vi "Initialize Sequence.vi"(8 "error in (no error)":errorcluster, 11 "Sequencer in":refnum<class "Sequencer.lvclass">) -> (0 "error out":errorcluster, 3 "Sequencer out":refnum<class "Sequencer.lvclass">)   [LabVIEW 2015, in "Sequencer.lvlib" / "Sequencer.lvclass"]
uses:
  Sequencer.lvclass
  IO Device/IO Device Messages/Set Global Channel Properties Msg/Set Global Channel Properties Msg.lvclass
  IO Device/IO Device Messages/SetAOTask Msg/SetAOTask Msg.lvclass
  SequencerConfig.lvclass
  SequencerInfo.lvclass
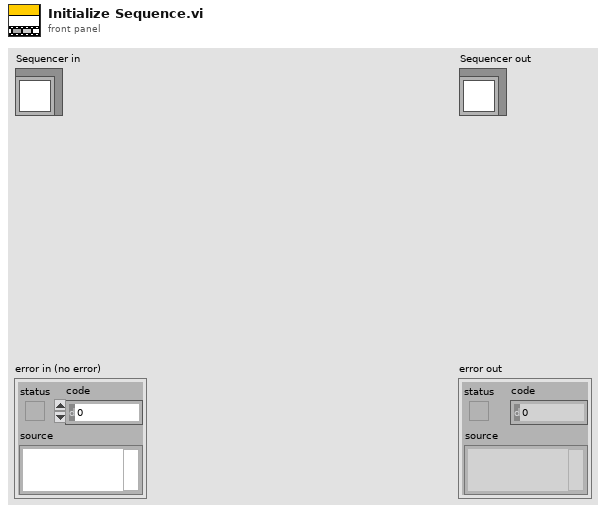
[diagram p1: front panel]
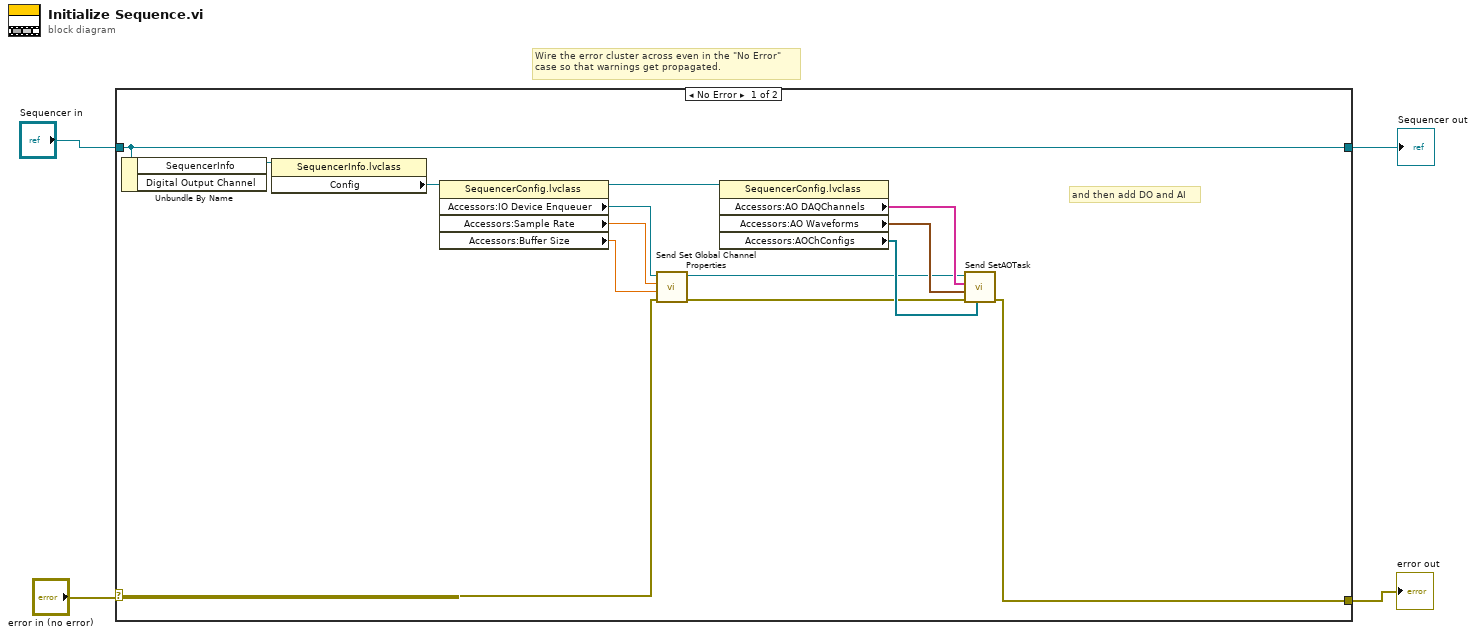
[diagram p0: block diagram]
diagram:
  # "Wire the error cluster across even in the \"No Error\"\ncase so that warnings get propagated."
  n1 = case shown="No Error" "error in (no error)" {
    selector: "error in (no error)" -> [w6 w20]
    tunnel: [w5 w20] -> w3
    tunnel: [w18 w19] -> w1
    tunnel: "Sequencer in" -> [w18 w19]
    frame No Error {
      # "and then add DO and AI"
      n2 = Unbundle By Name(w18) -> ("SequencerInfo"=w17:refnum<class "SequencerInfo.lvclass">)  [unwired: 1 out]
      n3 = property class="SequencerInfo.lvclass"(reference=w17) -> ("Config"=w16:refnum<class "SequencerConfig.lvclass">)  [unwired: 1 in, 2 out]
      n4 = property class="SequencerConfig.lvclass"(reference=w16) -> (reference out=w15:refnum<class "SequencerConfig.lvclass">, "Accessors:IO Device Enqueuer"=w14:refnum<class "Message Enqueuer.lvclass">, "Accessors:Sample Rate"=w13:dbl, "Accessors:Buffer Size"=w12:dbl)  [unwired: 1 in, 1 out]
      n5 = call "Send Set Global Channel Properties.vi"("error in (no error)"=w6, "Buffer Size"=w12, "Sample Rate"=w13, "Message Enqueuer in"=w14) -> ("error out"=w7:errorcluster, "Message Enqueuer out"=w8:refnum<class "Message Enqueuer.lvclass">)  [unwired: 6 in]
      n6 = property class="SequencerConfig.lvclass"(reference=w15) -> ("Accessors:AO DAQChannels"=w9:tag[], "Accessors:AO Waveforms"=w10:waveform(dbl)[], "Accessors:AOChConfigs"=w11:refnum<class "AOChConfig.lvclass">[])  [unwired: 1 in, 2 out]
      n7 = call "Send SetAOTask.vi"("AOChConfigs"=w11, "error in (no error)"=w7, "AO Waveforms"=w10, "AO DAQChannels"=w9, "Message Enqueuer in"=w8) -> ("error out"=w5:errorcluster)  [unwired: 5 in, 1 out]
    }
    frame Error {
    }
  }
  "error out" <- w3
  "Sequencer out" <- w1
